vi "Write multipage TIFF.vi"(7 "number of TIFF slices":i32, 8 "error in (no error)":errorcluster, 9 "cxd file handle":u32, 10 "offset":i32, 11 "TomoConversion in":refnum<class "TomoConversion.lvclass">) -> (0 "error out":errorcluster, 2 "TIFF file path":path, 3 "TomoConversion out":refnum<class "TomoConversion.lvclass">)   [LabVIEW 2012, in "TomoConversion.lvclass"]
uses:
  TomoConversion.lvclass
  dependencies/LabTIFF/LabTIFF/Opening Purpose.ctl
  TomoConversion.lvclass/TomoConversion.ctl
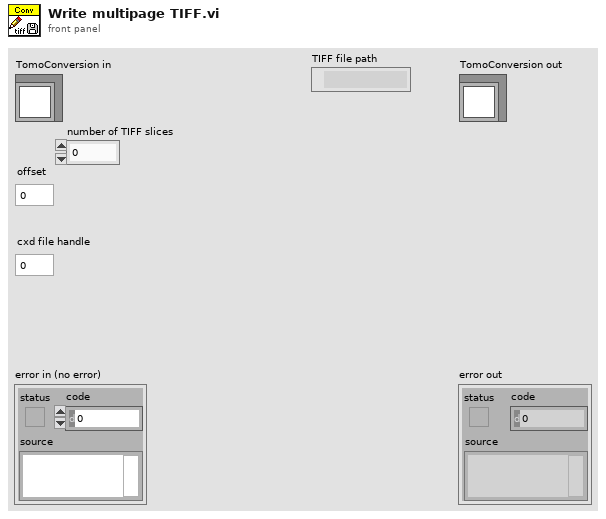
[diagram p1: front panel]
types:
  T1 = typedef "Opening Purpose.ctl" = enum16{"Read", "Write"}
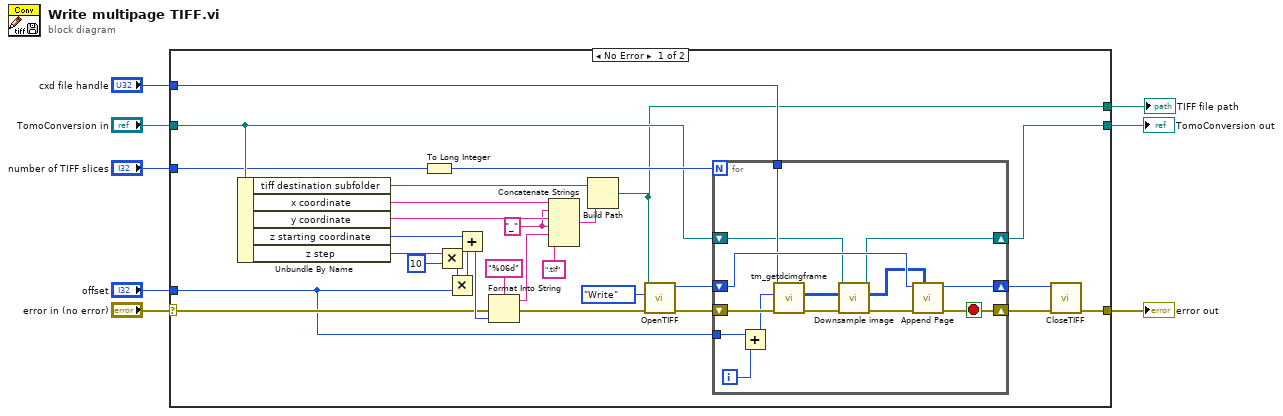
[diagram p0: block diagram]
diagram:
  n1 = case shown="No Error" "error in (no error)" {
    selector: "error in (no error)" -> [w30 w53]
    tunnel: [w11 w53] -> w7
    tunnel: [w14 w52] -> w5
    tunnel: "TomoConversion in" -> [w15 w52]
    tunnel: "offset" -> [w16 _]
    tunnel: "cxd file handle" -> [w18 _]
    tunnel: "number of TIFF slices" -> [w13 _]
    tunnel: [w9 _] -> w1
    frame No Error {
      w26 = "_"
      n2 = Unbundle By Name(w15) -> ("tiff destination subfolder"=w23:path, "x coordinate"=w28:string, "y coordinate"=w27:string, "z starting coordinate"=w33:i32, "z step"=w36:i32)
      n3 = To Long Integer(number=w13) -> (32bit integer=w17:i32)
      n4 = Multiply(x=w36, y=10) -> (x*y=w34:i32)
      n5 = Multiply(x=w34, y=w16) -> (x*y=w32:i32)
      n6 = Add(x=w33, y=w32) -> (x+y=w31:i32)
      n7 = Format Into String(format string="%06d", error in=w30, w31) -> (resulting string=w25:string, error out=w21:errorcluster)  [unwired: 1 in]
      n8 = Concatenate Strings(w28, w26, w27, w26, w25, ".tif") -> (w22:string)
      n9 = Build Path(base path=w23, name or relative path=w22) -> (appended path=w9:path)
      n10 = call "OpenTIFF.vi"("error in (no error)"=w21, "Opening Purpose"=Opening_Purpose."Write", "File Path"=w9) -> ("error out"=w20:errorcluster, "TIFF File Ref"=w19:i32)  [unwired: 7 in]
      n11 = for {
        N: w17 -> [_]
        shift-right: [w47] -> w12
        shift-left: w20 -> [w51]
        shift-right: [w49] -> w10
        shift-left: w19 -> [w50]
        tunnel: w18 -> [w48]
        tunnel: w16 -> [w46]
        shift-right: [w38] -> w14
        shift-left: w15 -> [w39]
        i -> [w45]
        stop <- w47 stop-if-true
        n12 = Add(x=w46, y=w45) -> (x+y=w44:i32)
        n13 = call <userlib>:"tm_getdcimgframe.vi"("error in (no error)"=w51, "Frame Index"=w44, "File Handle in"=w48) -> ("error out"=w43:errorcluster, "Data"=w41:u16[][])  [unwired: 5 in, 2 out]
        n14 = call-dynamic "Downsample image.vi"("error in (no error)"=w43, "Original image"=w41, "TomoConversion in"=w39) -> ("error out"=w42:errorcluster, "Downsampled image"=w40:u16[][], "TomoConversion out"=w38:refnum<class "TomoConversion.lvclass">)  [unwired: 6 in]
        n15 = call "Append Page.vi"("U16 Image"=w40, "error in (no error)"=w42, "TIFF File Ref"=w50) -> ("error out"=w47:errorcluster, "TIFF File Ref out"=w49:i32)  [unwired: 7 in]
      }
      n16 = call "CloseTIFF.vi"("error in (no error)"=w12, "TIFF File Ref"=w10) -> ("error out"=w11:errorcluster)  [unwired: 9 in]
    }
    frame Error {
    }
  }
  "error out" <- w7
  "TomoConversion out" <- w5
  "TIFF file path" <- w1
